vi "query setpoint ramping.vi"(8 "error in (no error)":errorcluster, 11 "VISA session":refnum<visa-resource-name>) -> (0 "error out":errorcluster, 2 "Setpoint Ramping?":bool, 3 "dup VISA session":refnum<visa-resource-name>)   [LabVIEW 2023]
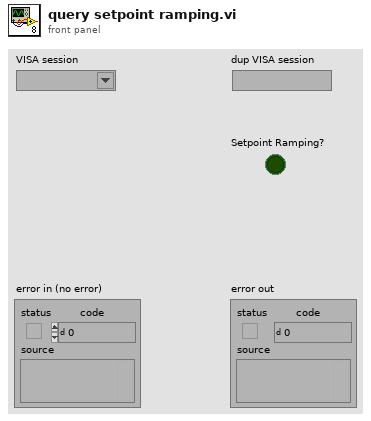
[diagram p1: front panel]
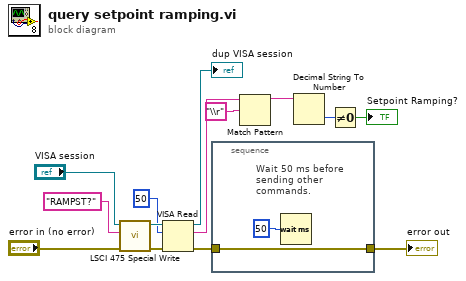
[diagram p0: block diagram]
diagram:
  n1 = call "LSCI 475 Special Write.vi"("error in (no error)"="error in (no error)", "Write Buffer (\"\")"="RAMPST?", "VISA session"="VISA session") -> ("error out"=w7:errorcluster, "dup VISA session"=w8:refnum<visa-resource-name>)  [unwired: 6 in, 1 out]
  n2 = VISA Read(VISA resource name=w8, byte count=u32 50, error in (no error)=w7) -> (VISA resource name out=→"dup VISA session":refnum<visa-resource-name>, read buffer=w5:string, error out=w3:errorcluster)  [unwired: 1 out]
  n3 = stacked-sequence {
    tunnel: w3 -> [w15]
    tunnel: [w15] -> w12
    frame #0 {
      # "Wait 50 ms before\nsending other\ncommands."
      n4 = Wait (ms)(milliseconds to wait=u32 50) -> ()  [unwired: 1 out]
    }
  }
  "error out" <- w12
  n5 = Match Pattern(string=w5, regular expression="\\r") -> (before substring=w1:string)  [unwired: 1 in, 3 out]
  n6 = Decimal String To Number(string=w1) -> (number=w9:i32)  [unwired: 2 in, 1 out]
  n7 = Not Equal To 0?(x=w9) -> (x != 0?=→"Setpoint Ramping?":bool)
